vi "GenerateWave.vi"(6 "Detune":dbl, 8 "NOTE":enum32{"BASS", "LOW MID", "MID", "HIGH", "LEAD"}(ring), 9 "WAVE TYPE":u16, 10 "DRIVE":dbl, 11 "SampleLenght":dbl) -> (3 "OUT":dbl[](array[numeric]))   [LabVIEW 2025]
uses:
  <vilib>/Analysis/NI_AALBase.lvlib
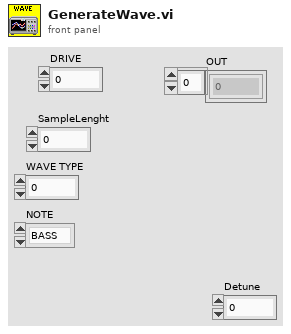
[diagram p1: front panel]
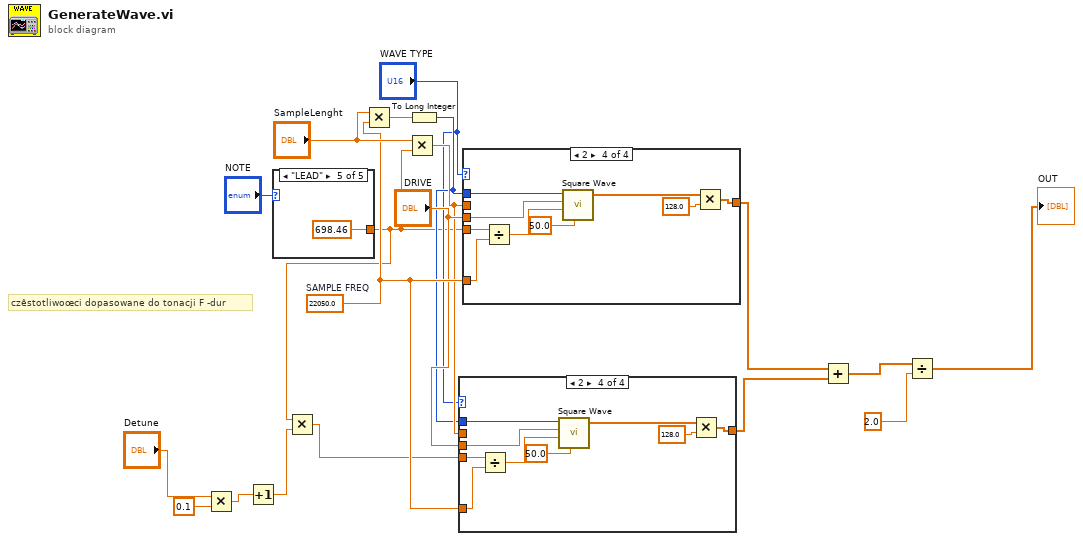
[diagram p0: block diagram]
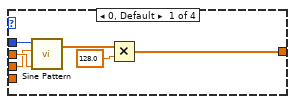
[diagram p2: hidden frame]
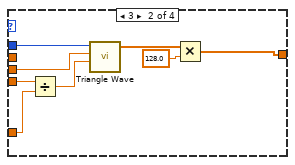
[diagram p3: hidden frame]
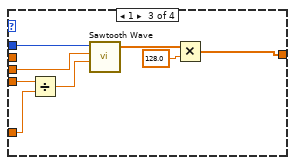
[diagram p4: hidden frame]
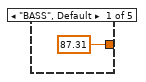
[diagram p5: hidden frame]
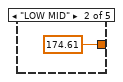
[diagram p6: hidden frame]
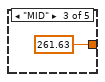
[diagram p7: hidden frame]
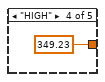
[diagram p8: hidden frame]
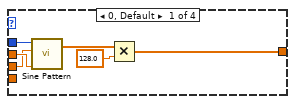
[diagram p9: hidden frame]
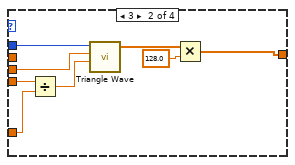
[diagram p10: hidden frame]
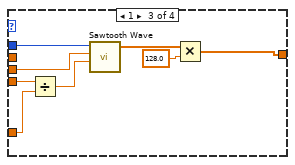
[diagram p11: hidden frame]
diagram:
  w16 = 22050.0  # SAMPLE FREQ
  # "czêstotliwoœci dopasowane do tonacji F -dur"
  n1 = Multiply(x="Detune", y=0.1) -> (x*y=w9:dbl)
  n2 = Increment(x=w9) -> (x+1=w7:dbl)
  n3 = case shown="\"LEAD\"" "NOTE" {
    tunnel: [87.31 ("cycles") 174.61 ("cycles") 261.63 ("cycles") 349.23 ("cycles") 698.46 ("cycles")] -> w8
    frame "BASS", Default {
    }
    frame "LOW MID" {
    }
    frame "MID" {
    }
    frame "HIGH" {
    }
    frame "LEAD" {
    }
  }
  n4 = Multiply(x=w8, y=w7) -> (x*y=w6:dbl)
  n5 = Multiply(x="SampleLenght", y=w16) -> (x*y=w17:dbl)
  n6 = Multiply(x="SampleLenght", y=w8) -> (x*y=w14:dbl)
  n7 = To Long Integer(number=w17) -> (32bit integer=w13:i32)
  n8 = case shown="2" "WAVE TYPE" {
    tunnel: [w26 w35 w43 w52] -> w4
    tunnel: w14 -> [w29 _ _ _]
    tunnel: "DRIVE" -> [w28 w37 w45 w55]
    tunnel: w13 -> [w27 w38 w46 w47]
    tunnel: w6 -> [_ w33 w41 w50]
    tunnel: w16 -> [_ w34 w42 w51]
    frame 0, Default {
      n9 = call <vilib>:"Sine Pattern.vi"("cycles"=w29, "amplitude"=w28, "samples"=w27) -> ("Sinusoidal Pattern"=w25:dbl[])  [unwired: 1 in, 1 out]
      n10 = Multiply(x=w25, y=128.0) -> (x*y=w26:dbl[])
    }
    frame 3 {
      n11 = Divide(x=w33, y=w34) -> (x/y=w32:dbl)
      n12 = call <vilib>:"Triangle Wave.vi"("samples"=w38, "amplitude"=w37, "frequency"=w32) -> ("triangle wave"=w31:dbl[])  [unwired: 2 in, 2 out]
      n13 = Multiply(x=w31, y=128.0) -> (x*y=w35:dbl[])
    }
    frame 1 {
      n14 = Divide(x=w41, y=w42) -> (x/y=w40:dbl)
      n15 = call <vilib>:"Sawtooth Wave.vi"("samples"=w46, "amplitude"=w45, "frequency"=w40) -> ("sawtooth wave"=w39:dbl[])  [unwired: 2 in, 2 out]
      n16 = Multiply(x=w39, y=128.0) -> (x*y=w43:dbl[])
    }
    frame 2 {
      n17 = Divide(x=w50, y=w51) -> (x/y=w49:dbl)
      n18 = call <vilib>:"Square Wave.vi"("samples"=w47, "amplitude"=w55, "frequency"=w49, "duty cycle (%)"=50.0) -> ("square wave"=w48:dbl[])  [unwired: 2 in, 2 out]
      n19 = Multiply(x=w48, y=128.0) -> (x*y=w52:dbl[])
    }
  }
  n20 = case shown="2" "WAVE TYPE" {
    tunnel: [w57 w66 w74 w83] -> w5
    tunnel: w14 -> [w60 _ _ _]
    tunnel: "DRIVE" -> [w59 w68 w76 w86]
    tunnel: w13 -> [w58 w69 w77 w78]
    tunnel: w8 -> [_ w64 w72 w81]
    tunnel: w16 -> [_ w65 w73 w82]
    frame 0, Default {
      n21 = call <vilib>:"Sine Pattern.vi"("cycles"=w60, "amplitude"=w59, "samples"=w58) -> ("Sinusoidal Pattern"=w56:dbl[])  [unwired: 1 in, 1 out]
      n22 = Multiply(x=w56, y=128.0) -> (x*y=w57:dbl[])
    }
    frame 3 {
      n23 = Divide(x=w64, y=w65) -> (x/y=w63:dbl)
      n24 = call <vilib>:"Triangle Wave.vi"("samples"=w69, "amplitude"=w68, "frequency"=w63) -> ("triangle wave"=w62:dbl[])  [unwired: 2 in, 2 out]
      n25 = Multiply(x=w62, y=128.0) -> (x*y=w66:dbl[])
    }
    frame 1 {
      n26 = Divide(x=w72, y=w73) -> (x/y=w71:dbl)
      n27 = call <vilib>:"Sawtooth Wave.vi"("samples"=w77, "amplitude"=w76, "frequency"=w71) -> ("sawtooth wave"=w70:dbl[])  [unwired: 2 in, 2 out]
      n28 = Multiply(x=w70, y=128.0) -> (x*y=w74:dbl[])
    }
    frame 2 {
      n29 = Divide(x=w81, y=w82) -> (x/y=w80:dbl)
      n30 = call <vilib>:"Square Wave.vi"("samples"=w78, "amplitude"=w86, "frequency"=w80, "duty cycle (%)"=50.0) -> ("square wave"=w79:dbl[])  [unwired: 2 in, 2 out]
      n31 = Multiply(x=w79, y=128.0) -> (x*y=w83:dbl[])
    }
  }
  n32 = Add(x=w5, y=w4) -> (x+y=w3:dbl[])
  n33 = Divide(x=w3, y=2.0) -> (x/y=→"OUT":dbl[])
